vi "Write Header - GUI Data.vi"(8 "error in (no error)":errorcluster, 11 "Save Image in":refnum<class "Save Image.lvclass">) -> (0 "error out":errorcluster, 3 "Save Image out":refnum<class "Save Image.lvclass">)   [LabVIEW 2018, in "Save Image.lvclass"]
uses:
  Save Image.lvclass
  Save Image.lvclass/Save Image.ctl
  TCS_ACS/TCS_ACS.lvclass
  Simulated_Header/Simulated_Header.lvclass
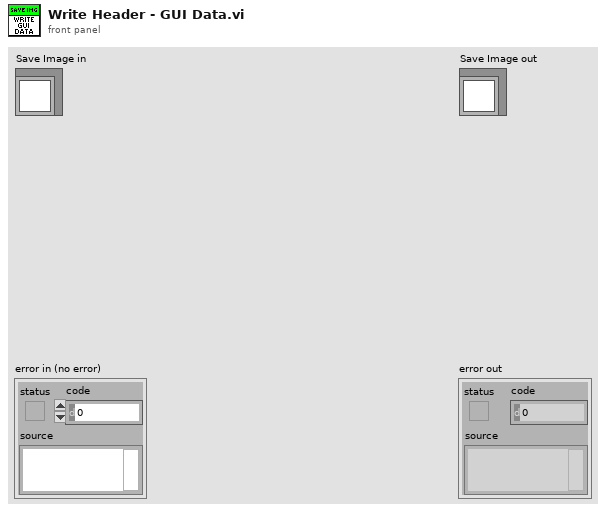
[diagram p1: front panel]
types:
  T1 = cluster{"OBJ":string, "RA":string, "DEC":string, "EPOCH":dbl, "AIRMASS":dbl, "JD":dbl, "SD":string, "HA":string, "DATEOBS":string, "FOCUS":string, "WS_DEFAULT":string, "TEMP":string, "BAR":string, "HUM":string, "FILTER":string, "CTRLINTE":string, "TCSDATE":string}
  T2 = cluster{"FILENAME":cluster{"Name":string, "Value":string, "Comment":string}, "OBSERVER":cluster{"Name":string, "Value":string, "Comment":string}, "PROGRID":cluster{"Name":string, "Value":string, "Comment":string}, "OBJECT":cluster{"Name":string, "Value":string, "Comment":string}, "NIGHTDIR":cluster{"Name":string, "Value":string, "Comment":string}, "CHANNEL":cluster{"Name":string, "Value":string, "Comment":string}, "INSTRUME":cluster{"Name":string, "Value":string, "Comment":string}, "NEXPSEQ":cluster{"Name":string, "Value":u16, "Comment":string}, "SEQINDEX":cluster{"Name":string, "Value":u16, "Comment":string}, "OBSTYPE":cluster{"Name":string, "Value":string, "Comment":string}, "READMOD":cluster{"Name":string, "Value":string, "Comment":string}, "READMODE":cluster{"Name":string, "Value":string, "Comment":string}, "ACQMODE":cluster{"Name":string, "Value":string, "Comment":string}, "PREAMP":cluster{"Name":string, "Value":string, "Comment":string}, "READOUT":cluster{"Name":string, "Value":string, "Comment":string}, "VSHIFT":cluster{"Name":string, "Value":string, "Comment":string}, "TRIGGER":cluster{"Name":string, "Value":string, "Comment":string}, "EMMODE":cluster{"Name":string, "Value":string, "Comment":string}, "EMGAIN":cluster{"Name":string, "Value":u16, "Comment":string}, "VBIN":cluster{"Name":string, "Value":u16, "Comment":string}, "HBIN":cluster{"Name":string, "Value":u16, "Comment":string}, "INITLIN":cluster{"Name":string, "Value":u16, "Comment":string}, "INITCOL":cluster{"Name":string, "Value":u16, "Comment":string}, "FINALLIN":cluster{"Name":string, "Value":u16, "Comment":string}, "FINALCOL":cluster{"Name":string, "Value":u16, "Comment":string}, "KSERLEN":cluster{"Name":string, "Value":u16, "Comment":string}, "SHUTTER":cluster{"Name":string, "Value":string, "Comment":string}, "OPENSHT":cluster{"Name":string, "Value":u16, "Comment":string}, "CLOSESHT":cluster{"Name":string, "Value":u16, "Comment":string}, "DATE":cluster{"Name":string, "Value":string, "Comment":string}, "GAIN":cluster{"Name":string, "Value":dbl, "Comment":string}, "GAINERR":cluster{"Name":string, "Value":dbl, "Comment":string}, "RDNOISE":cluster{"Name":string, "Value":dbl, "Comment":string}, "RNOISERR":cluster{"Name":string, "Value":dbl, "Comment":string}, "SKYFIBER":cluster{"Name":string, "Value":string, "Comment":string}, "CALFIBER":cluster{"Name":string, "Value":string, "Comment":string}, "UTDATE":cluster{"Name":string, "Value":string, "Comment":string}, "LOCTIME":cluster{"Name":string, "Value":string, "Comment":string}, "MJD":cluster{"Name":string, "Value":dbl, "Comment":string}, "OBSLON":cluster{"Name":string, "Value":string, "Comment":string}, "OBSLAT":cluster{"Name":string, "Value":string, "Comment":string}, "OBSALT":cluster{"Name":string, "Value":dbl, "Comment":string}, "EXPTIME":cluster{"Name":string, "Value":dbl, "Comment":string}, "TELRA":cluster{"Name":string, "Value":string, "Comment":string}, "TELDEC":cluster{"Name":string, "Value":string, "Comment":string}, "RA":cluster{"Name":string, "Value":string, "Comment":string}, "DEC":cluster{"Name":string, "Value":string, "Comment":string}, "RA_DEG":cluster{"Name":string, "Value":dbl, "Comment":string}, "DEC_DEG":cluster{"Name":string, "Value":dbl, "Comment":string}, "EPOCH":cluster{"Name":string, "Value":dbl, "Comment":string}, "HA":cluster{"Name":string, "Value":string, "Comment":string}, "HAD":cluster{"Name":string, "Value":dbl, "Comment":string}, "AIRMASS":cluster{"Name":string, "Value":dbl, "Comment":string}, "AMSTART":cluster{"Name":string, "Value":dbl, "Comment":string}, "AMEND":cluster{"Name":string, "Value":dbl, "Comment":string}, "XOFFSET":cluster{"Name":string, "Value":dbl, "Comment":string}, "YOFFSET":cluster{"Name":string, "Value":dbl, "Comment":string}, "PA":cluster{"Name":string, "Value":dbl, "Comment":string}, "CAMFOC":cluster{"Name":string, "Value":string, "Comment":string}, "TELFOC":cluster{"Name":string, "Value":dbl, "Comment":string}, "TCSUT":cluster{"Name":string, "Value":string, "Comment":string}, "TCSST":cluster{"Name":string, "Value":string, "Comment":string}, "MOONDIST":cluster{"Name":string, "Value":dbl, "Comment":string}, "MOONALT":cluster{"Name":string, "Value":dbl, "Comment":string}, "MOONPHAS":cluster{"Name":string, "Value":string, "Comment":string}, "ADC":cluster{"Name":string, "Value":string, "Comment":string}, "ADCSPEED":cluster{"Name":string, "Value":dbl, "Comment":string}, "CALMIRR":cluster{"Name":string, "Value":string, "Comment":string}, "GUIDING":cluster{"Name":string, "Value":string, "Comment":string}, "GUIDTEXP":cluster{"Name":string, "Value":dbl, "Comment":string}, "GUIDFREQ":cluster{"Name":string, "Value":dbl, "Comment":string}, "GUIDOBJX":cluster{"Name":string, "Value":dbl, "Comment":string}, "GUIDOBJY":cluster{"Name":string, "Value":dbl, "Comment":string}, "AVGYCORR":cluster{"Name":string, "Value":dbl, "Comment":string}, "AVGXCORR":cluster{"Name":string, "Value":dbl, "Comment":string}, "GFOCUS":cluster{"Name":string, "Value":dbl, "Comment":string}, "THARLAMP":cluster{"Name":string, "Value":string, "Comment":string}, "HALLAMP":cluster{"Name":string, "Value":string, "Comment":string}, "AGITATOR":cluster{"Name":string, "Value":string, "Comment":string}, "THARMIRR":cluster{"Name":string, "Value":string, "Comment":string}, "DSTATUS":cluster{"Name":string, "Value":string, "Comment":string}, "DPOS":cluster{"Name":string, "Value":dbl, "Comment":string}, "DTEMP":cluster{"Name":string, "Value":dbl, "Comment":string}, "DHUM":cluster{"Name":string, "Value":string, "Comment":string}, "DLAMP":cluster{"Name":string, "Value":string, "Comment":string}, "DFLAT":cluster{"Name":string, "Value":string, "Comment":string}, "TEMPEXT":cluster{"Name":string, "Value":string, "Comment":string}, "PRESSURE":cluster{"Name":string, "Value":string, "Comment":string}, "HUMIDITY":cluster{"Name":string, "Value":string, "Comment":string}, "WINDDIR":cluster{"Name":string, "Value":string, "Comment":string}, "WINSPEED":cluster{"Name":string, "Value":dbl, "Comment":string}, "SHTTTL":cluster{"Name":string, "Value":string, "Comment":string}, "COOLER":cluster{"Name":string, "Value":string, "Comment":string}, "TEMP":cluster{"Name":string, "Value":i16, "Comment":string}, "TEMPST":cluster{"Name":string, "Value":string, "Comment":string}, "SERN":cluster{"Name":string, "Value":u16, "Comment":string}, "COMMENT":cluster{"Name":string, "Value":string, "Comment":string}, "BITPIX":cluster{"Name":string, "Value":u16, "Comment":string}, "EXTEND":cluster{"Name":string, "Value":string, "Comment":string}, "FRAME_T":cluster{"Name":string, "Value":string, "Comment":string}, "VCLOCK":cluster{"Name":string, "Value":string, "Comment":string}, "ADCHNNL":cluster{"Name":string, "Value":u16, "Comment":string}, "JD":cluster{"Name":string, "Value":dbl, "Comment":string}, "SD":cluster{"Name":string, "Value":string, "Comment":string}, "FILTER":cluster{"Name":string, "Value":string, "Comment":string}, "ACSVRSN":cluster{"Name":string, "Value":string, "Comment":string}, "CTRLINTER":cluster{"Name":string, "Value":string, "Comment":string}, "TCSDATE":cluster{"TCSDATE":string, "Value":string, "Comment":string}}
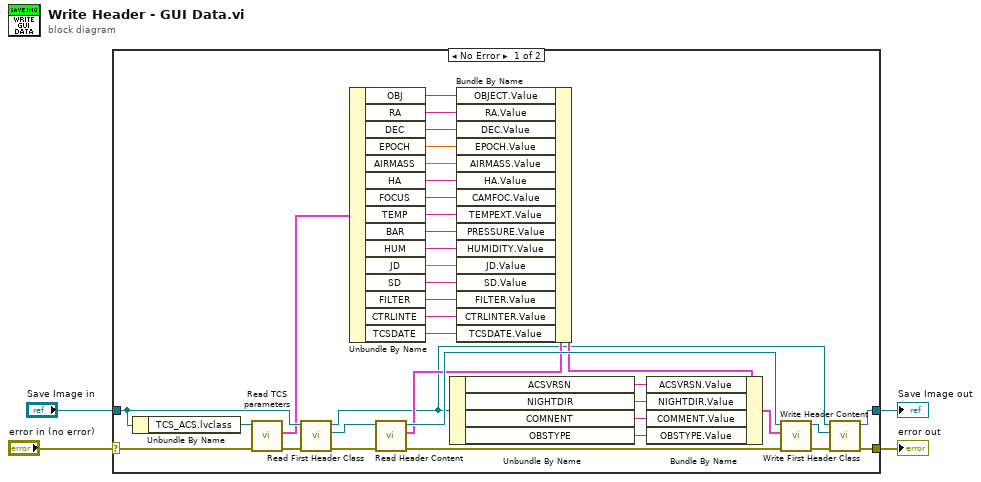
[diagram p0: block diagram]
diagram:
  n1 = case shown="No Error" "error in (no error)" {
    selector: "error in (no error)" -> [w15 w41]
    tunnel: [w40 w41] -> w3
    tunnel: [w39 w42] -> w1
    tunnel: "Save Image in" -> [w38 w42]
    frame No Error {
      n2 = Unbundle By Name(w38) -> ("TCS_ACS.lvclass"=w37:refnum<class "TCS_ACS.lvclass">)
      n3 = call "Read TCS parameters.vi"("error in (no error)"=w15, "TCS_ACS in"=w37) -> ("error out"=w14:errorcluster, "TCS parameters"=w36:T1)  [unwired: 7 in, 1 out]
      n4 = call "Read First Header Class.vi"("error in (no error)"=w14, "Save Image in"=w38) -> ("error out"=w28:errorcluster, "Simulated_Header.lvclass"=w29:refnum<class "Simulated_Header.lvclass">, "Save Image out"=w8:refnum<class "Save Image.lvclass">)  [unwired: 7 in]
      n5 = Unbundle By Name(w36) -> ("OBJ"=w35:string, "RA"=w34:string, "DEC"=w33:string, "EPOCH"=w32:dbl, "AIRMASS"=w31:dbl, "HA"=w30:string, "FOCUS"=w23:string, "TEMP"=w22:string, "BAR"=w21:string, "HUM"=w20:string, "JD"=w19:dbl, "SD"=w18:string, "FILTER"=w17:string, "CTRLINTE"=w6:string, "TCSDATE"=w5:string)
      n6 = call "Read Header Content.vi"("error in (no error)"=w28, "Simulated_Header in"=w29) -> ("error out"=w25:errorcluster, "Header Content"=w16:T2, "Simulated_Header out"=w24:refnum<class "Simulated_Header.lvclass">)  [unwired: 7 in]
      n7 = Unbundle By Name(w8) -> ("ACSVRSN"=w7:string, "NIGHTDIR"=w11:string, "COMNENT"=w10:string, "OBSTYPE"=w9:string)
      n8 = Bundle By Name(cluster=w16, "OBJECT.Value"=w35, "RA.Value"=w34, "DEC.Value"=w33, "EPOCH.Value"=w32, "AIRMASS.Value"=w31, "HA.Value"=w30, "CAMFOC.Value"=w23, "TEMPEXT.Value"=w22, "PRESSURE.Value"=w21, "HUMIDITY.Value"=w20, "JD.Value"=w19, "SD.Value"=w18, "FILTER.Value"=w17, "CTRLINTER.Value"=w6, "TCSDATE.Value"=w5) -> (w13:T2)
      n9 = Bundle By Name(cluster=w13, "ACSVRSN.Value"=w7, "NIGHTDIR.Value"=w11, "COMMENT.Value"=w10, "OBSTYPE.Value"=w9) -> (w12:T2)
      n10 = call "Write Header Content.vi"("error in (no error)"=w25, "Header Content"=w12, "Simulated_Header in"=w24) -> ("error out"=w26:errorcluster, "Simulated_Header out"=w27:refnum<class "Simulated_Header.lvclass">)  [unwired: 7 in]
      n11 = call "Write First Header Class.vi"("error in (no error)"=w26, "Simulated_Header.lvclass"=w27, "Save Image in"=w8) -> ("error out"=w40:errorcluster, "Save Image out"=w39:refnum<class "Save Image.lvclass">)  [unwired: 7 in]
    }
    frame Error {
    }
  }
  "error out" <- w3
  "Save Image out" <- w1
